vi "DSF.Engine.Memory.Cache.Set Transfers Groups.vi"(10 "Transfers Groups":refnum<class "DSF.Engine.Transfer Group.lvclass">[](array[class]), 11 "Cache in":refnum<class "DSF.Engine.Memory.Cache.lvclass">) -> (3 "Cache out":refnum<class "DSF.Engine.Memory.Cache.lvclass">)   [LabVIEW 2017, in "DSF.Engine.lvlib" / "DSF.Engine.Memory.Cache.lvclass"]
uses:
  DSF.Engine.Memory.Cache.lvclass
  Transfer/DSF.Engine.Transfer Group.lvclass
  DSF.Engine.Memory.Cache.lvclass/DSF.Engine.Memory.Cache.ctl
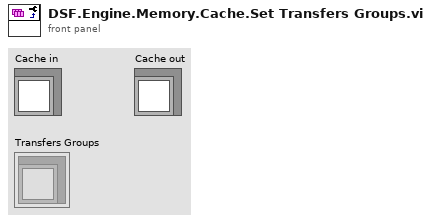
[diagram p1: front panel]
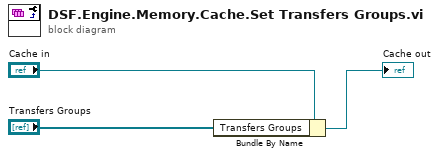
[diagram p0: block diagram]
diagram:
  n1 = Bundle By Name(cluster="Cache in", "Transfers Groups"="Transfers Groups") -> (→"Cache out":refnum<class "DSF.Engine.Memory.Cache.lvclass">)
